vi "number_to_sring.vi"(11 "Numeric":dbl format="%#_8g") -> (2 "result string":string)   [LabVIEW 2015]
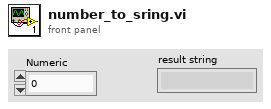
[diagram p1: front panel]
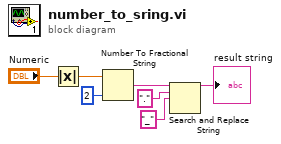
[diagram p0: block diagram]
diagram:
  n1 = Absolute Value(x="Numeric") -> (abs(x)=w4:dbl)
  n2 = Number To Fractional String(number=w4, precision (6)=i16 2) -> (F-format string=w3:string)  [unwired: 2 in]
  n3 = Search and Replace String(input string=w3, search string=".", replace string="_" ("replace string (\"\")")) -> (result string=→"result string":string)  [unwired: 5 in, 3 out]
